vi "image_pixel calib_once (SubVI).vi"() -> (1 "Y posiiton on image \n(pattern detection)":sgl, 2 "X posiiton on image \n(pattern detection)":sgl)   [LabVIEW 2014]
doc: "Detect stuck bead pattern to get slide drift information."
uses:
  Global 1 extract image.vi
panel:
  in  "BCG Values":T1={"Brightness"=200.0, "Contrast"=50.0, "Gamma"=1.0}
  in  "adjust constrast?":bool
  in  "Remaining Inputs":T2={"Circle Descriptor (Shape Detection 1)"={"Min Radius"=3.0, "Max Radius"=500.0}, "Y Scale.Mapping Mode (Line Profile 1)"=0}
  in  "Match Options (Shape Detection 1)":T3={"Rotation"=TRUE, "Scale"=FALSE, "Occlusion"=FALSE, "Range Settings"=[{"Match Constraints"=0, "Min"=0.0, "Max"=360.0}]} {"Range Settings"."Match Constraints" items=["Rotation Angle (degrees)", "Scale Factor (%)", "Occlusion (%)"]}
  in  "Minimum match score (Shape Detection 1)":dbl=800.0
  in  "Curve Parameters (Shape Detection 1)":T4={"Extraction Mode"=0, "Edge Threshold"=11, "Edge Filter Size"=1, "Min Length"=1, "Row Search Step Size"=1, "Col Search Step Size"=1, "Max Endpoint Gap"=1, "Closed"=FALSE, "Subpixel"=FALSE} {"Extraction Mode" items=["Normal", "Uniform Regions"]; "Edge Filter Size" items=["Fine", "Normal"]}
  in  "ROI Descriptor (Shape Detection 1)":T5={"Global Rectangle"=[6, 17, 113, 117], "Contours"=[{"ID"=enum."External", "Type"=3, "Coordinates"=[6, 17, 113, 117]}]} {"Contours"."Type" items=["No Selection", "Point", "Line", "Rectangle", "Oval", "Polygon", "Freehand Region", "Annulus", "Unused2", "Unused3", "Broken Line", "Freehand Line", "Rotated Rectangle"]}
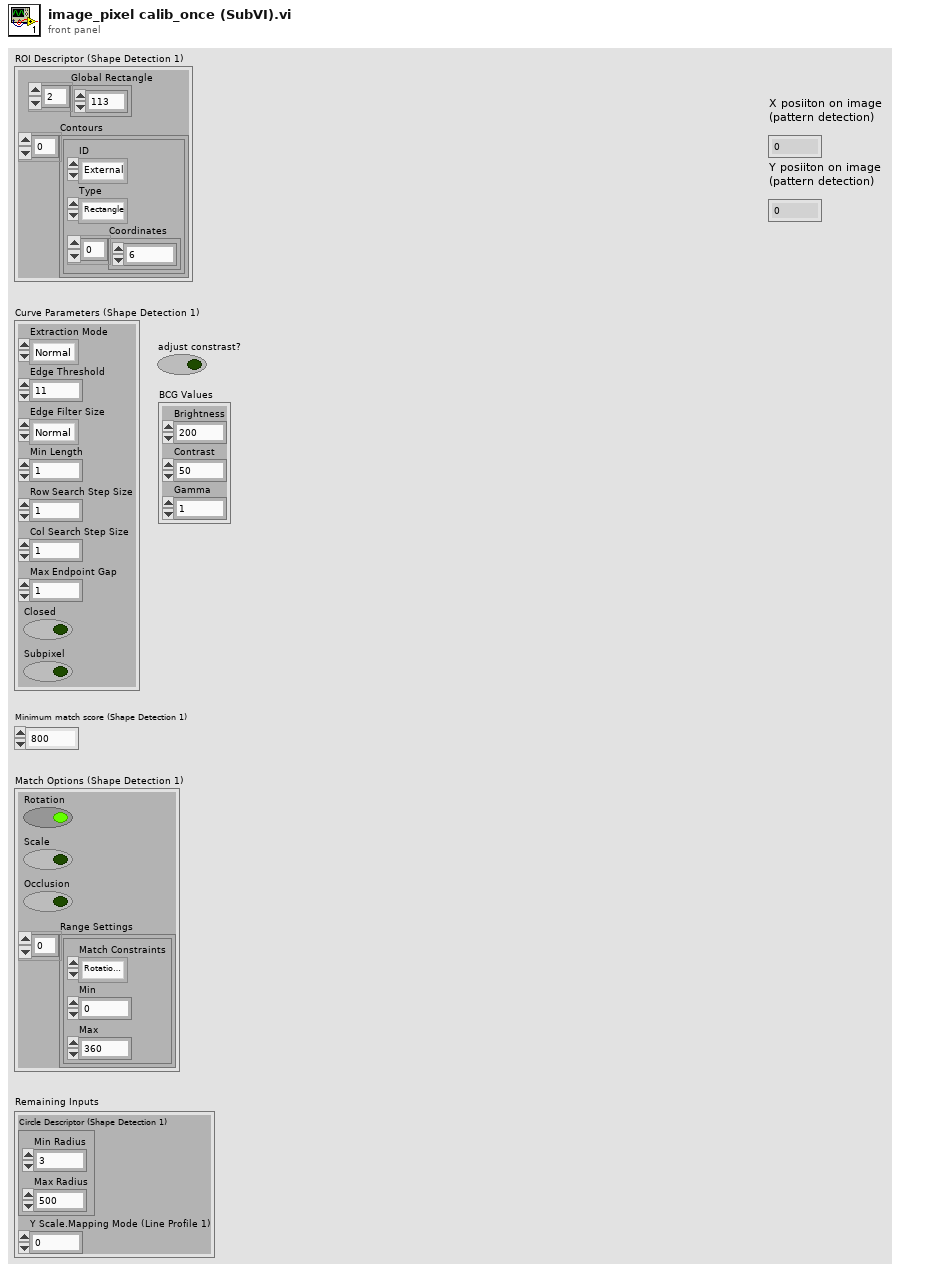
[diagram p1: front panel]
types:
  T1 = cluster{"Brightness":sgl, "Contrast":sgl, "Gamma":sgl}
  T2 = cluster{"Circle Descriptor (Shape Detection 1)":cluster{"Min Radius":dbl, "Max Radius":dbl}, "Y Scale.Mapping Mode (Line Profile 1)":u8}
  T3 = cluster{"Rotation":bool, "Scale":bool, "Occlusion":bool, "Range Settings":cluster{"Match Constraints":u32, "Min":dbl, "Max":dbl}[]}
  T4 = cluster{"Extraction Mode":u32, "Edge Threshold":i32, "Edge Filter Size":u32, "Min Length":i32, "Row Search Step Size":i32, "Col Search Step Size":i32, "Max Endpoint Gap":i32, "Closed":bool, "Subpixel":bool}
  T5 = cluster{"Global Rectangle":i32[], "Contours":cluster{"ID":enum32{"External", "Internal"}, "Type":u32, "Coordinates":i32[]}[]}
  T6 = typedef "IMAQ Image.ctl" = refnum<image>
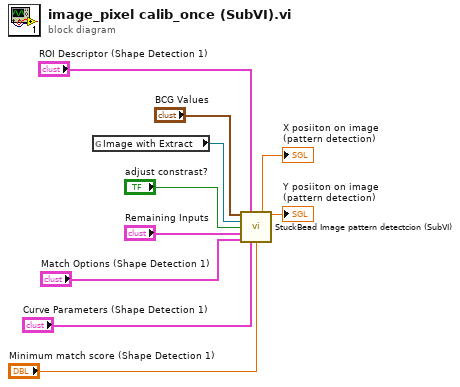
[diagram p0: block diagram]
diagram:
  n1 = global read "Global 1 extract image.vi" "Image with Extract"() -> (w3:T6)
  n2 = call "StuckBead Image pattern detectcion (SubVI).vi"("BCG Values"="BCG Values", "ROI Descriptor (Shape Detection 1)"="ROI Descriptor (Shape Detection 1)", "Refnum in"=w3, "adjust?"="adjust constrast?", "Remaining Inputs"="Remaining Inputs", "Match Options (Shape Detection 1)"="Match Options (Shape Detection 1)", "Curve Parameters (Shape Detection 1)"="Curve Parameters (Shape Detection 1)", "Minimum match score (Shape Detection 1)"="Minimum match score (Shape Detection 1)") -> ("X posiiton on image \n(pattern detection)"=→"X posiiton on image \n(pattern detection)":sgl, "Y posiiton on image \n(pattern detection)"=→"Y posiiton on image \n(pattern detection)":sgl)  [unwired: 6 out]
